vi "ExSubCloseCamUnInit.vi"(1 "error in (no error)":errorcluster, 2 "Camera Handle":u32) -> (0 "error out":errorcluster)   [LabVIEW 2010]
panel:
  # "ExSubCloseCamUnInit:\nThis SubVI closes the camera and\ncalls UnLoad to close the Toolkit."
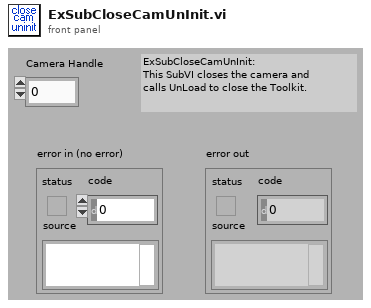
[diagram p1: front panel]
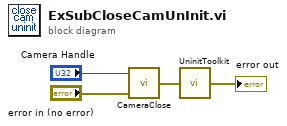
[diagram p0: block diagram]
diagram:
  n1 = call <userlib>:"CameraClose.vi"("error in"="error in (no error)", "Camera Handle"="Camera Handle") -> ("error out"=w2:errorcluster)
  n2 = call <userlib>:"UninitToolkit.vi"("error in"=w2) -> ("error out"=→"error out":errorcluster)
